vi "cmd_scan.vi"(8 "error in (no error)":errorcluster, 11 "JSON":string) -> (0 "error out":errorcluster)   [LabVIEW 2021]
doc: "Command template VI.\n\nWhen you want to create a new command, please copy and modify this VI.\nThe command vi should aPerform a simple x-y scan.\n\n :param nx: Specifies the number of data point x\n :param ny: Specifies the number of data point y\n :param lx: Specifies the length along x\n :param ly: Specifies the length along y\n :param cx: Specifies the center position x\n :param cy: Specifies the center position y\n :param avg: Specifies the averaged count for each data pointbe placed in the host/cmd directory."
uses:
  fpga/fpga_dtype_scan_config.ctl
  fpga/fpga_dtype_sgl_8ch.ctl
  fpga/fpga_dtype_index.ctl
panel:
  in  "args":T1
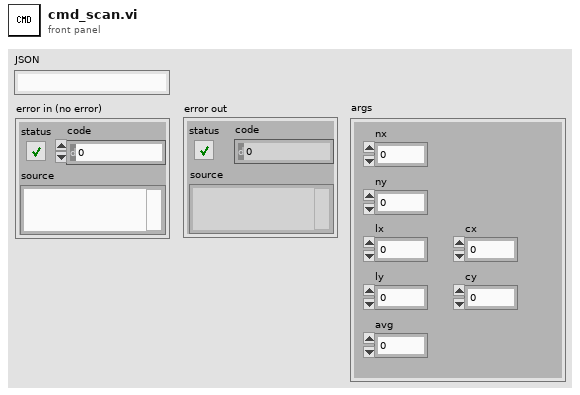
[diagram p1: front panel]
types:
  T1 = cluster{"nx":i32, "ny":i32, "lx":sgl, "ly":sgl, "avg":i32, "cx":sgl, "cy":sgl}
  T2 = typedef "fpga_dtype_index.ctl" = cluster{"page":i16, "2nd":i16, "1st":i16}
  T3 = typedef "fpga_dtype_sgl_8ch.ctl" = cluster{"ch 0":sgl, "ch 1":sgl, "ch 2":sgl, "ch 3":sgl, "ch 4":sgl, "ch 5":sgl, "ch 6":sgl, "ch 7":sgl}
  T4 = typedef "fpga_dtype_scan_config.ctl" = cluster{"data points":i16, "average counts":i16, "delta per point":T3, "bidirectional scan":bool, "auto reversal":bool}
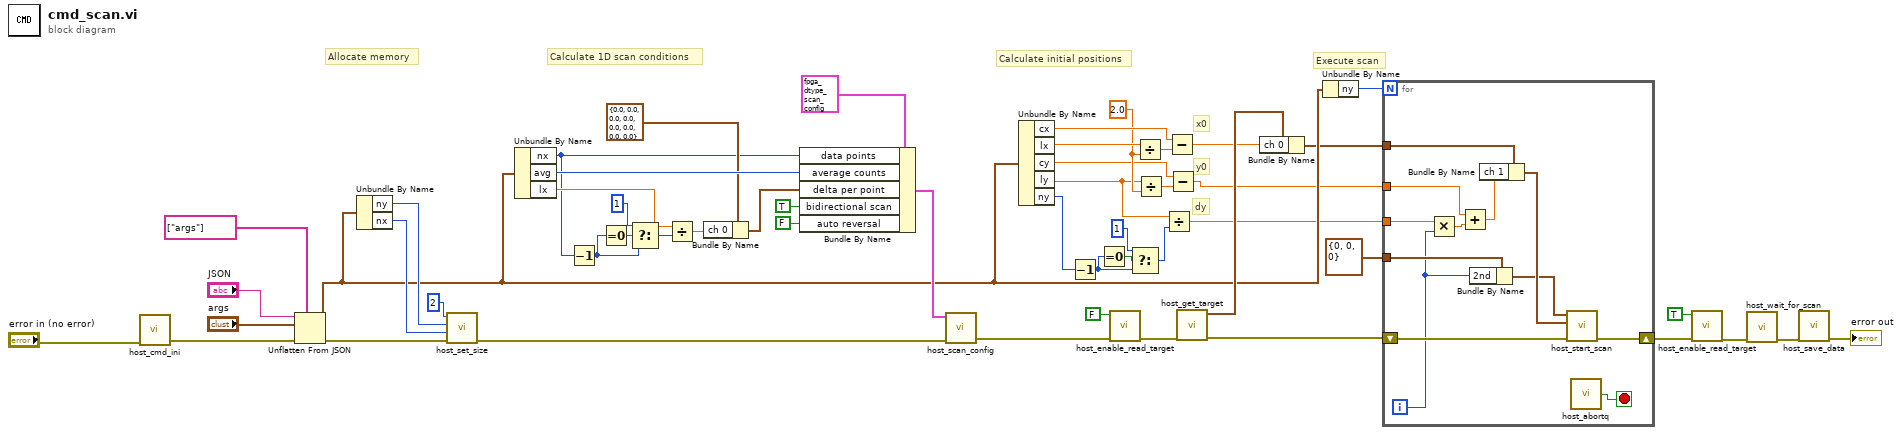
[diagram p0: block diagram]
diagram:
  w36 = sgl 2.0 ("y")
  # "Execute scan"
  # "Allocate memory"
  # "dy"
  # "y0"
  # "x0"
  # "Calculate initial positions"
  # "Calculate 1D scan conditions"
  n1 = call "host_cmd_ini.vi"("error in (no error)"="error in (no error)") -> ("error out"=w8:errorcluster)  [unwired: 10 in]
  n2 = Unflatten From JSON(path=string[] ["args"], JSON string="JSON", type and defaults="args", error in (no error)=w8) -> (value=w26:T1, error out=w33:errorcluster)  [unwired: 3 in]
  n3 = Unbundle By Name(w26) -> ("ny"=w30:i32, "nx"=w29:i32)
  n4 = call "host_set_size.vi"("error in (no error)"=w33, "fast"=w29, "slow"=w30, "page"=2) -> ("error out"=w32:errorcluster)  [unwired: 7 in]
  n5 = Unbundle By Name(w26) -> ("nx"=w19:i32, "avg"=w45:i32, "lx"=w44:sgl)
  n6 = Decrement(x=w19) -> (x-1=w10:i32)
  n7 = Equal To 0?(x=w10) -> (x = 0?=w11:bool)
  n8 = Select(t=1, s=w11, f=w10) -> (s? t:f=w17:i32)
  n9 = Divide(x=w44, y=w17) -> (x/y=w42:sgl)
  n10 = Bundle By Name(cluster=T3 {"ch 0"=0.0, "ch 1"=0.0, "ch 2"=0.0, "ch 3"=0.0, "ch 4"=0.0, "ch 5"=0.0, "ch 6"=0.0, "ch 7"=0.0} ("delta per point"), "ch 0"=w42) -> (w41:T3)
  n11 = Bundle By Name(cluster=T4 {"data points"=0, "average counts"=0, "delta per point"={"ch 0"=0.0, "ch 1"=0.0, "ch 2"=0.0, "ch 3"=0.0, "ch 4"=0.0, "ch 5"=0.0, "ch 6"=0.0, "ch 7"=0.0}, "bidirectional scan"=FALSE, "auto reversal"=FALSE} ("scan config"), "data points"=w19, "average counts"=w45, "delta per point"=w41, "bidirectional scan"=TRUE, "auto reversal"=FALSE) -> (w48:T4)
  n12 = call "host_scan_config.vi"("error in"=w32, "scan config"=w48) -> ("error out"=w1:errorcluster)  [unwired: 9 in]
  n13 = Unbundle By Name(w26) -> ("cx"=w38:sgl, "lx"=w40:sgl, "cy"=w35:sgl, "ly"=w34:sgl, "ny"=w15:i32)
  n14 = Decrement(x=w15) -> (x-1=w12:i32)
  n15 = Equal To 0?(x=w12) -> (x = 0?=w13:bool)
  n16 = call "host_enable_read_target.vi"("error in"=w1, "enable read target?"=FALSE) -> ("error out"=w2:errorcluster)  [unwired: 9 in]
  n17 = Select(t=1, s=w13, f=w12) -> (s? t:f=w14:i32)
  n18 = Divide(x=w40, y=w36) -> (x/y=w39:sgl)
  n19 = Divide(x=w34, y=w36) -> (x/y=w37:sgl)
  n20 = Divide(x=w34, y=w14) -> (x/y=w22:sgl)
  n21 = Subtract(x=w38, y=w39) -> (x-y=w27:sgl)
  n22 = Subtract(x=w35, y=w37) -> (x-y=w21:sgl)
  n23 = call "host_get_target.vi"("error in"=w2) -> ("error out"=w23:errorcluster, "target"=w28:T3)  [unwired: 9 in]
  n24 = Bundle By Name(cluster=w28, "ch 0"=w27) -> (w24:T3)
  n25 = Unbundle By Name(w26) -> ("ny"=w25:i32)
  n26 = for {
    N: w25 -> [_]
    tunnel: w24 -> [w61]
    shift-right: [w63] -> w4
    shift-left: w23 -> [w64]
    tunnel: w22 -> [w55]
    tunnel: w21 -> [w62]
    tunnel: T2 {"page"=0, "2nd"=0, "1st"=0} ("index offset") -> [w58]
    i -> [w54]
    stop <- w65 stop-if-true
    n27 = Multiply(x=w55, y=w54) -> (x*y=w56:sgl)
    n28 = Add(x=w62, y=w56) -> (x+y=w60:sgl)
    n29 = Bundle By Name(cluster=w58, "2nd"=w54) -> (w57:T2)
    n30 = Bundle By Name(cluster=w61, "ch 1"=w60) -> (w59:T3)
    n31 = call "host_start_scan.vi"("error in"=w64, "initial positions"=w59, "index offset"=w57) -> ("error out"=w63:errorcluster)  [unwired: 6 in, 2 out]
    n32 = call "host_abortq.vi"() -> ("abort"=w65:bool)  [unwired: 1 in]
  }
  n33 = call "host_enable_read_target.vi"("error in"=w4, "enable read target?"=TRUE) -> ("error out"=w5:errorcluster)  [unwired: 9 in]
  n34 = call "host_wait_for_scan.vi"("error in (no error)"=w5) -> ("error out"=w9:errorcluster)  [unwired: 10 in]
  n35 = call "host_save_data.vi"("error in"=w9) -> ("error out"=→"error out":errorcluster)  [unwired: 10 in]
